vi "InclinometerTest.vi"() -> ()   [LabVIEW 2016]
uses:
  <vilib>/FPGAPlugInAG/cRIO-9038/niLvFpga_Open_cRIO-9038.vi
  <vilib>/rvi/interface/common/dynamic/niFpgaDynamicAddResources.vi
  <vilib>/FPGAPlugInAG/Dynamic/niLvFpga_Abort_Dynamic.vi
  <vilib>/FPGAPlugInAG/Dynamic/niLvFpga_Reset_Dynamic.vi
  <vilib>/FPGAPlugInAG/Dynamic/niLvFpga_Run_Dynamic.vi
  <vilib>/Utility/error.llb/Error Cluster From Error Code.vi
  <vilib>/rvi/errors/niLvFpgaAdjustHostInterfaceError.vi
  <vilib>/FPGAPlugInAG/Dynamic/niLvFpga_Close_Dynamic.vi
  <vilib>/rvi/interface/nirviOpenFPGA/nirviOpenFPGA.xnode
  FPGA Bitfiles/Modbus_FPGATarget_Inclinometer_RQMDSPMx2Gg.lvbitx
  Inclinometer.vi
  <vilib>/rvi/interface/nirviMethod/nirviMethod.xnode
  <vilib>/rvi/interface/nirviCloseFPGA/nirviCloseFPGA.xnode
  <vilib>/rvi/errors/niLvFpgaMergeErrorWithErrorCode.vi
  <vilib>/FPGAPlugInAG/Dynamic/niLvFpga_ReadFifo_Dynamic.vi
panel:
  in  "Boolean":bool
  in  "Send":bool
  out "Output":u8[](array[numeric]) format="%02x"
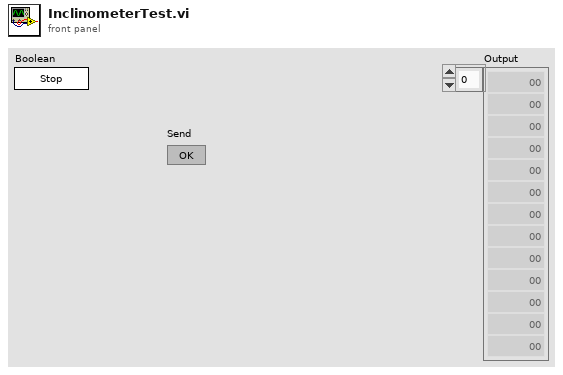
[diagram p1: front panel]
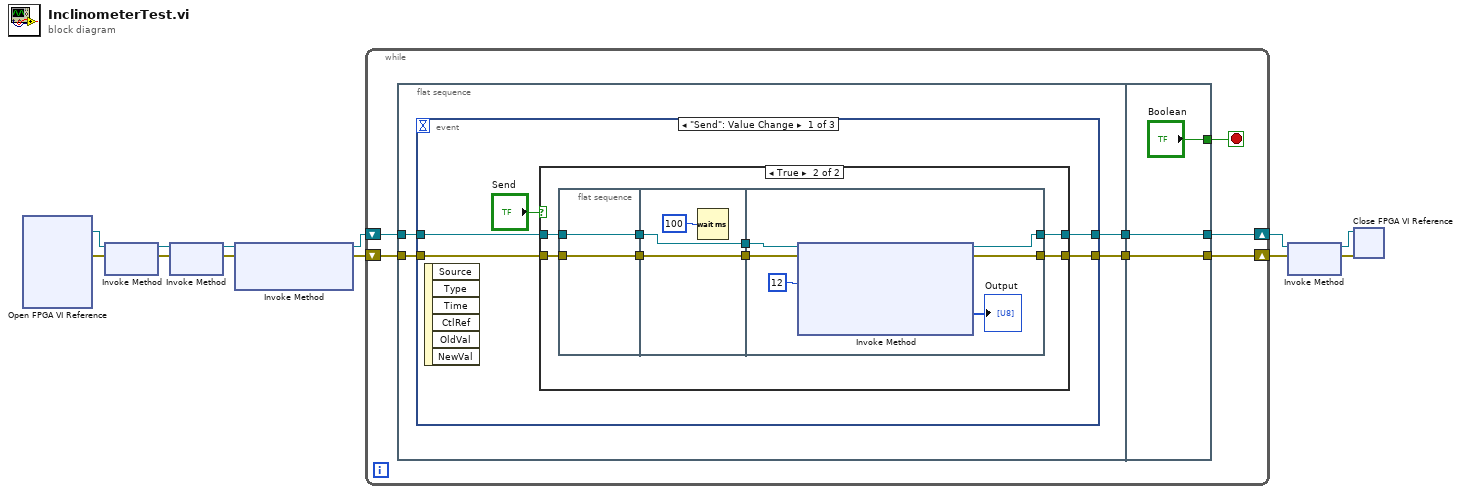
[diagram p0: block diagram]
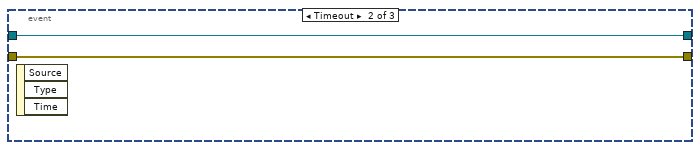
[diagram p3: hidden frame]
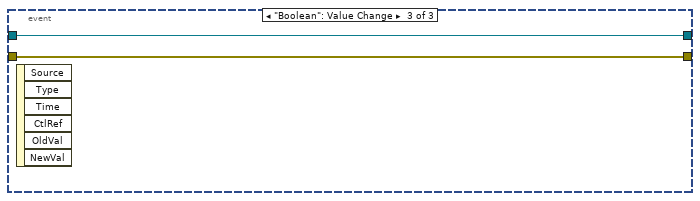
[diagram p4: hidden frame]
diagram:
  n1 = xnode "Open FPGA VI Reference"() -> ("FPGA VI Reference Out"=w12:refnum<k20>, "error out"=w7:errorcluster)  [unwired: 2 in]
  n2 = xnode "Invoke Method"("FPGA VI Reference In"=w12, "error in"=w7) -> ("FPGA VI Reference Out"=w11:refnum<k20>, "error out"=w8:errorcluster)
  n3 = xnode "Invoke Method"("FPGA VI Reference In"=w11, "error in"=w8) -> ("FPGA VI Reference Out"=w10:refnum<k20>, "error out"=w9:errorcluster)
  n4 = xnode "Invoke Method"("FPGA VI Reference In"=w10, "error in"=w9) -> ("FPGA VI Reference Out"=w6:refnum<k20>, "error out"=w5:errorcluster)  [unwired: 1 in]
  n5 = while {
    shift-right: [w17] -> w4
    shift-left: w6 -> [w19]
    shift-right: [w16] -> w3
    shift-left: w5 -> [w18]
    stop <- w13 stop-if-true
    n6 = flat-sequence {
      tunnel: w19 -> [w23]
      tunnel: w18 -> [w22]
      tunnel: [w21] -> w15
      tunnel: [w20] -> w14
      tunnel: [w55] -> w16
      tunnel: [w56] -> w17
      tunnel: w15 -> [w56]
      tunnel: w14 -> [w55]
      tunnel: ["Boolean"] -> w13
      frame #0 {
        n7 = event shown="[0] \"Send\": Value Change" {
          selector: _ -> [_ _ _]
          dyn-events: _ -> [_ _ _]
          timeout: _ -> [_ _ _]
          tunnel: w23 -> [w28 w51 w53]
          tunnel: w22 -> [w27 w50 w52]
          tunnel: [w26 w51 w53] -> w21
          tunnel: [w25 w50 w52] -> w20
          event "Send": Value Change {
            n8 = event-data() -> ()  [unwired: 1 in, 6 out]
            n9 = case shown="True" "Send" {
              tunnel: w28 -> [w30 w38]
              tunnel: w27 -> [w29 w37]
              tunnel: [w30 w36] -> w26
              tunnel: [w29 w35] -> w25
              frame False {
              }
              frame True {
                n10 = flat-sequence {
                  tunnel: w38 -> [w39]
                  tunnel: w37 -> [w40]
                  tunnel: [w40] -> w33
                  tunnel: [w39] -> w32
                  tunnel: [w42] -> w34
                  tunnel: w33 -> [w42]
                  tunnel: w32 -> [w41]
                  tunnel: [w41] -> w31
                  tunnel: [w49] -> w36
                  tunnel: [w48] -> w35
                  tunnel: w34 -> [w47]
                  tunnel: w31 -> [w46]
                  frame #0 {
                  }
                  frame #1 {
                    n11 = Wait (ms)(milliseconds to wait=u32 100) -> ()  [unwired: 1 out]
                  }
                  frame #2 {
                    n12 = xnode "Invoke Method"("FPGA VI Reference In"=w46, "error in"=w47, "Number of Elements"=u32 12) -> ("FPGA VI Reference Out"=w49:refnum<k20>, "error out"=w48:errorcluster, "Data"=→"Output":u8[])  [unwired: 1 in, 1 out]
                  }
                }
              }
            }
          }
          event Timeout {
            n13 = event-data() -> ()  [unwired: 1 in, 3 out]
          }
          event "Boolean": Value Change {
            n14 = event-data() -> ()  [unwired: 1 in, 6 out]
          }
        }
      }
      frame #1 {
      }
    }
  }
  n15 = xnode "Invoke Method"("FPGA VI Reference In"=w4, "error in"=w3) -> ("FPGA VI Reference Out"=w2:refnum<k20>, "error out"=w1:errorcluster)
  n16 = xnode "Close FPGA VI Reference"("FPGA VI Reference In"=w2, "error in"=w1) -> ()  [unwired: 1 out]
